vi "SP_SetZTheta.vi"(4 "Move Z?":bool, 5 "Move Theta?":bool, 6 "Theta Speed (10-100%)":dbl, 7 "Z Speed (10-100%)":dbl, 8 "error in (no error)":errorcluster, 9 "Theta in mdeg":dbl, 10 "Z in um":dbl, 11 "SemiProbe in":refnum<class "SemiProbe.lvclass">) -> (0 "error out":errorcluster, 3 "SemiProbe out":refnum<class "SemiProbe.lvclass">)   [LabVIEW 2019, in "SemiProbe.lvclass"]
uses:
  SemiProbe.lvclass
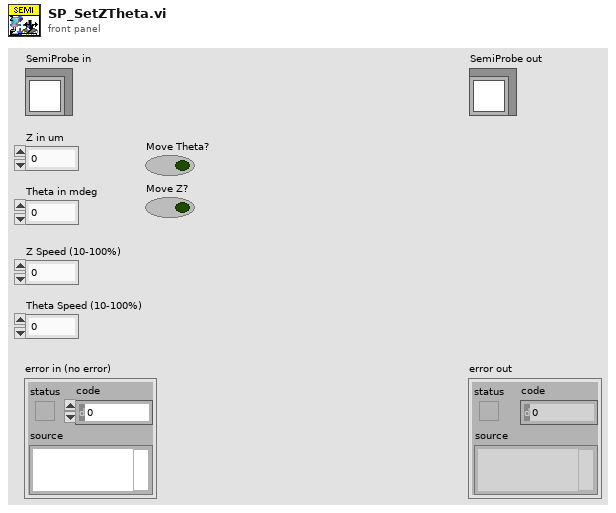
[diagram p1: front panel]
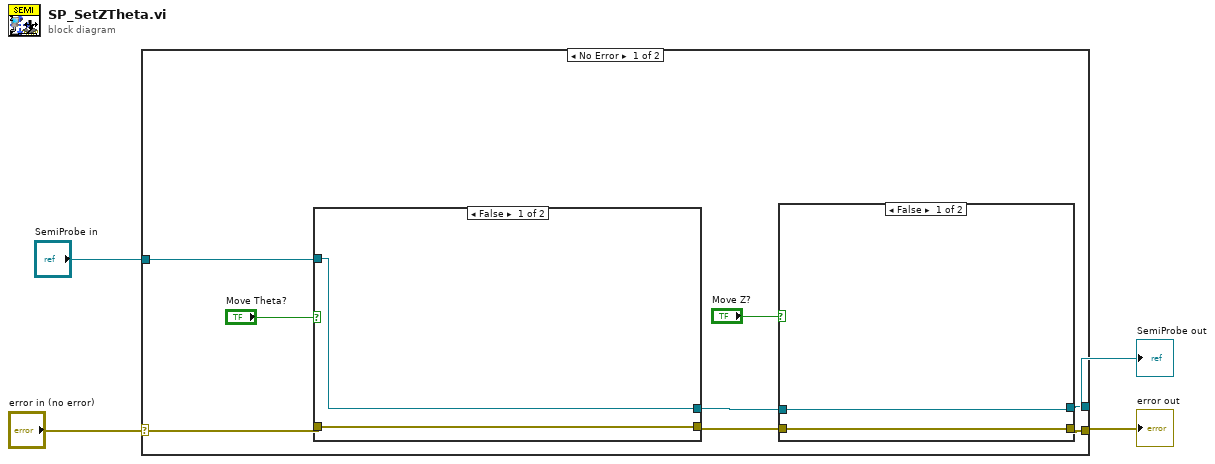
[diagram p0: block diagram]
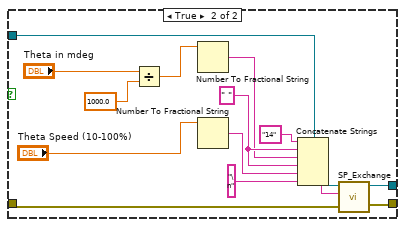
[diagram p2: hidden frame]
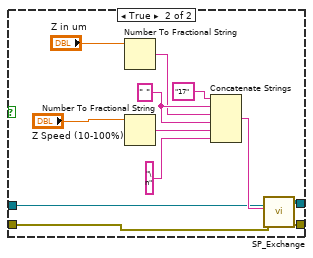
[diagram p3: hidden frame]
diagram:
  n1 = case shown="No Error" "error in (no error)" {
    selector: "error in (no error)" -> [w10 w44]
    tunnel: [w11 w44] -> w3
    tunnel: [w12 w43] -> w1
    tunnel: "SemiProbe in" -> [w9 w43]
    frame No Error {
      n2 = case shown="False" "Move Theta?" {
        tunnel: w10 -> [w13 w19]
        tunnel: w9 -> [w14 w17]
        tunnel: [w13 w16] -> w8
        tunnel: [w14 w15] -> w7
        frame False {
        }
        frame True {
          w25 = " "
          n3 = Divide(x="Theta in mdeg", y=1000.0) -> (x/y=w20:dbl)
          n4 = Number To Fractional String(number=w20) -> (F-format string=w23:string)  [unwired: 3 in]
          n5 = Number To Fractional String(number="Theta Speed (10-100%)") -> (F-format string=w24:string)  [unwired: 3 in]
          n6 = Concatenate Strings("14", w25, w23, w25, w24, "\n") -> (w18:string)
          n7 = call-dynamic "SP_Exchange.vi"("error in (no error)"=w19, "command"=w18, "SemiProbe in"=w17) -> ("error out"=w16:errorcluster, "SemiProbe out"=w15:refnum<class "SemiProbe.lvclass">)  [unwired: 4 in, 3 out]
        }
      }
      n8 = case shown="False" "Move Z?" {
        tunnel: [w30 w35] -> w12
        tunnel: [w29 w34] -> w11
        tunnel: w8 -> [w29 w32]
        tunnel: w7 -> [w30 w31]
        frame False {
        }
        frame True {
          w42 = " "
          n9 = Number To Fractional String(number="Z in um") -> (F-format string=w41:string)  [unwired: 3 in]
          n10 = Number To Fractional String(number="Z Speed (10-100%)") -> (F-format string=w37:string)  [unwired: 3 in]
          n11 = Concatenate Strings("17", w42, w41, w42, w37, "\n") -> (w33:string)
          n12 = call-dynamic "SP_Exchange.vi"("error in (no error)"=w32, "command"=w33, "SemiProbe in"=w31) -> ("error out"=w34:errorcluster, "SemiProbe out"=w35:refnum<class "SemiProbe.lvclass">)  [unwired: 4 in, 3 out]
        }
      }
    }
    frame Error {
    }
  }
  "error out" <- w3
  "SemiProbe out" <- w1
